vi "Get Single Plot Style.vi"(8 "Error In":errorcluster, 9 "index":i32, 11 "Plot Style in":T1) -> (0 "Error Out":errorcluster, 3 "Plot Style out":T2)   [LabVIEW 2019]
uses:
  Single Plot Style 2.ctl
  Plot Style 3.ctl
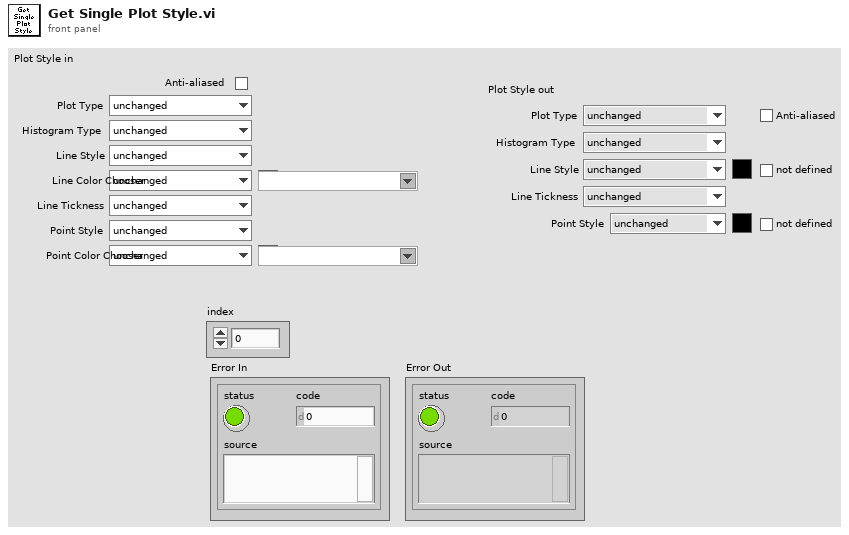
[diagram p1: front panel]
types:
  T1 = typedef "Plot Style 3.ctl" = cluster{"Plot Style":enum16{"unchanged", "Line", "Symbol", "Line + Symbol", "Histogram", "Histogram + Symbol"}, "Histogram Type":enum16{"unchanged", "Left Bound", "Center", "Right Bound"}, "Line Tickness":enum16{"unchanged", "Thin", "1 pixel", "2 pixel", "3 pixel", "4 pixel", "5 pixel"}, "Line Style":enum16{"unchanged", "Plain", "Long Dash", "Short Dash", "Long-Short Dash", "Long-Short-Short Dash"}, "Point Style":enum16{"unchanged", "None", "Empty Circle", "Filled Circle", "Thick Circle", "Dotted Circle", "Empty Square", "Filled Square", "Thick Square", "Dotted Square", "Small Filled Square", "Dot", "Cross", "Tiny Cross", "Large X", "Small x", "Diamond", "Small Empty Square"}, "Line Color":u32, "Point Color":u32, "Anti-aliased":bool, "Line Color Chooser":enum16{"unchanged", "Color Box", "Color List"}, "Point Color Chooser":enum16{"unchanged", "Color Box", "Color List"}, "Line Color List":string, "Point Color List":string}
  T2 = typedef "Single Plot Style 2.ctl" = cluster{"Plot Style":enum16{"unchanged", "Line", "Symbol", "Line + Symbol", "Histogram", "Histogram + Symbol"}, "Histogram Type":enum16{"unchanged", "Left Bound", "Center", "Right Bound"}, "Line Tickness":enum16{"unchanged", "Thin", "1 pixel", "2 pixel", "3 pixel", "4 pixel", "5 pixel"}, "Line Style":enum16{"unchanged", "Plain", "Long Dash", "Short Dash", "Long-Short Dash", "Long-Short-Short Dash"}, "Point Style":enum16{"unchanged", "None", "Empty Circle", "Filled Circle", "Thick Circle", "Dotted Circle", "Empty Square", "Filled Square", "Thick Square", "Dotted Square", "Small Filled Square", "Dot", "Cross", "Tiny Cross", "Large X", "Small x", "Diamond", "Small Empty Square"}, "Line Color":u32, "Line Color defined?":bool, "Point Color":u32, "Point Color defined?":bool, "Anti-aliased":bool}
  T3 = enum16{"unchanged", "Line", "Symbol", "Line + Symbol", "Histogram", "Histogram + Symbol"}
  T4 = enum16{"unchanged", "Left Bound", "Center", "Right Bound"}
  T5 = enum16{"unchanged", "Thin", "1 pixel", "2 pixel", "3 pixel", "4 pixel", "5 pixel"}
  T6 = enum16{"unchanged", "Plain", "Long Dash", "Short Dash", "Long-Short Dash", "Long-Short-Short Dash"}
  T7 = enum16{"unchanged", "None", "Empty Circle", "Filled Circle", "Thick Circle", "Dotted Circle", "Empty Square", "Filled Square", "Thick Square", "Dotted Square", "Small Filled Square", "Dot", "Cross", "Tiny Cross", "Large X", "Small x", "Diamond", "Small Empty Square"}
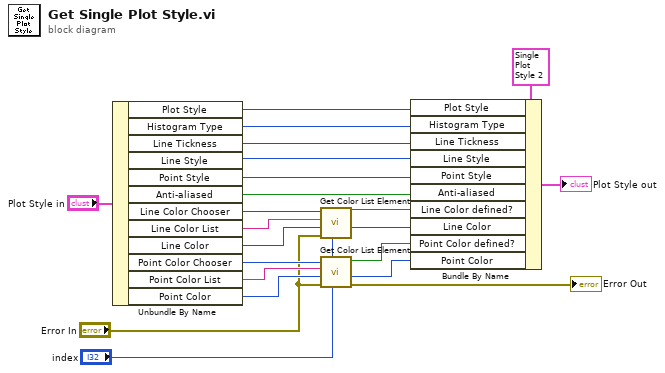
[diagram p0: block diagram]
diagram:
  n1 = Unbundle By Name("Plot Style in") -> ("Plot Style"=w19:T3, "Histogram Type"=w18:T4, "Line Tickness"=w17:T5, "Line Style"=w16:T6, "Point Style"=w15:T7, "Anti-aliased"=w14:bool, "Line Color Chooser"=w13:enum16{"unchanged", "Color Box", "Color List"}, "Line Color List"=w12:string, "Line Color"=w11:u32, "Point Color Chooser"=w8:enum16{"unchanged", "Color Box", "Color List"}, "Point Color List"=w7:string, "Point Color"=w6:u32)
  n2 = call "Get Color List Element.vi"("index"="index", "Error In"="Error In", "Color"=w11, "Color List"=w12, "Color Chooser"=w13) -> ("Color"=w9:u32, "Color defined?"=w10:bool)  [unwired: 4 in, 1 out]
  n3 = call "Get Color List Element.vi"("index"="index", "Error In"="Error In", "Color"=w6, "Color List"=w7, "Color Chooser"=w8) -> ("Error Out"=→"Error Out":errorcluster, "Color"=w4:u32, "Color defined?"=w5:bool)  [unwired: 4 in]
  n4 = Bundle By Name(cluster=T2 {"Plot Style"=enum."unchanged", "Histogram Type"=enum."unchanged", "Line Tickness"=enum."unchanged", "Line Style"=enum."unchanged", "Point Style"=enum."unchanged", "Line Color"=0, "Line Color defined?"=FALSE, "Point Color"=0, "Point Color defined?"=FALSE, "Anti-aliased"=FALSE} ("Plot Style out"), "Plot Style"=w19, "Histogram Type"=w18, "Line Tickness"=w17, "Line Style"=w16, "Point Style"=w15, "Anti-aliased"=w14, "Line Color defined?"=w10, "Line Color"=w9, "Point Color defined?"=w5, "Point Color"=w4) -> (→"Plot Style out":T2)
